vi "KML-Compose2.vi"(0 "TimerIN (sh)":u32, 1 "WriteToFile?":bool, 3 "SPD":string, 4 "path to vi or exe":path, 5 "ALT":string, 6 "HED":string, 7 "Range":string="1500", 9 "Tilt":string="0", 11 "error in":errorcluster, 12 "Current Location":string, 13 "Heading":string="0", 14 "Coords":string) -> (10 "Timer OUT (sh)":u32, 15 "error out":errorcluster)   [LabVIEW 8.6]
panel:
  out "resulting string":string
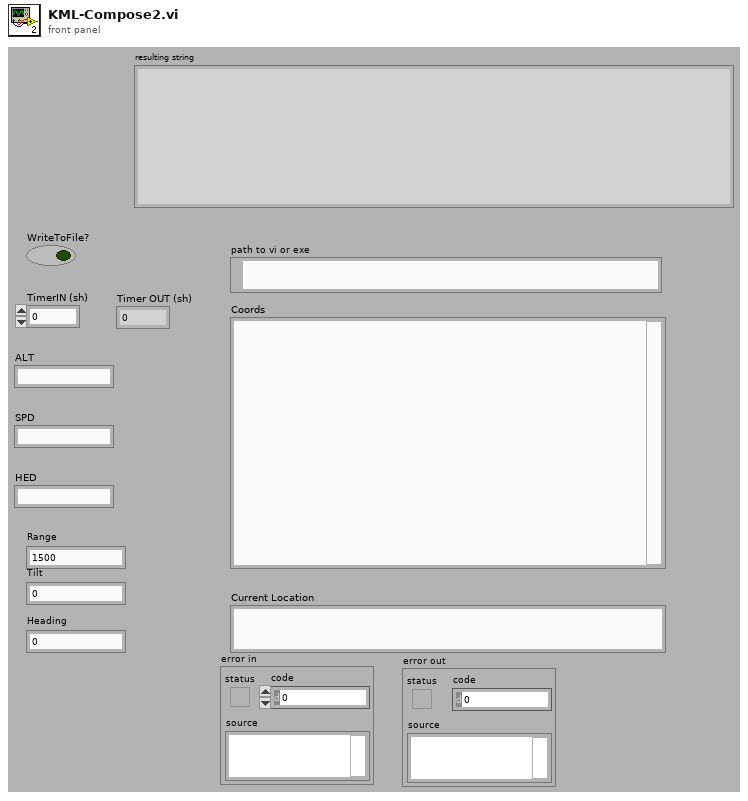
[diagram p1: front panel]
types:
  T1 = enum16{"open", "replace", "create", "open or create", "replace or create", "replace or create with confirmation"}
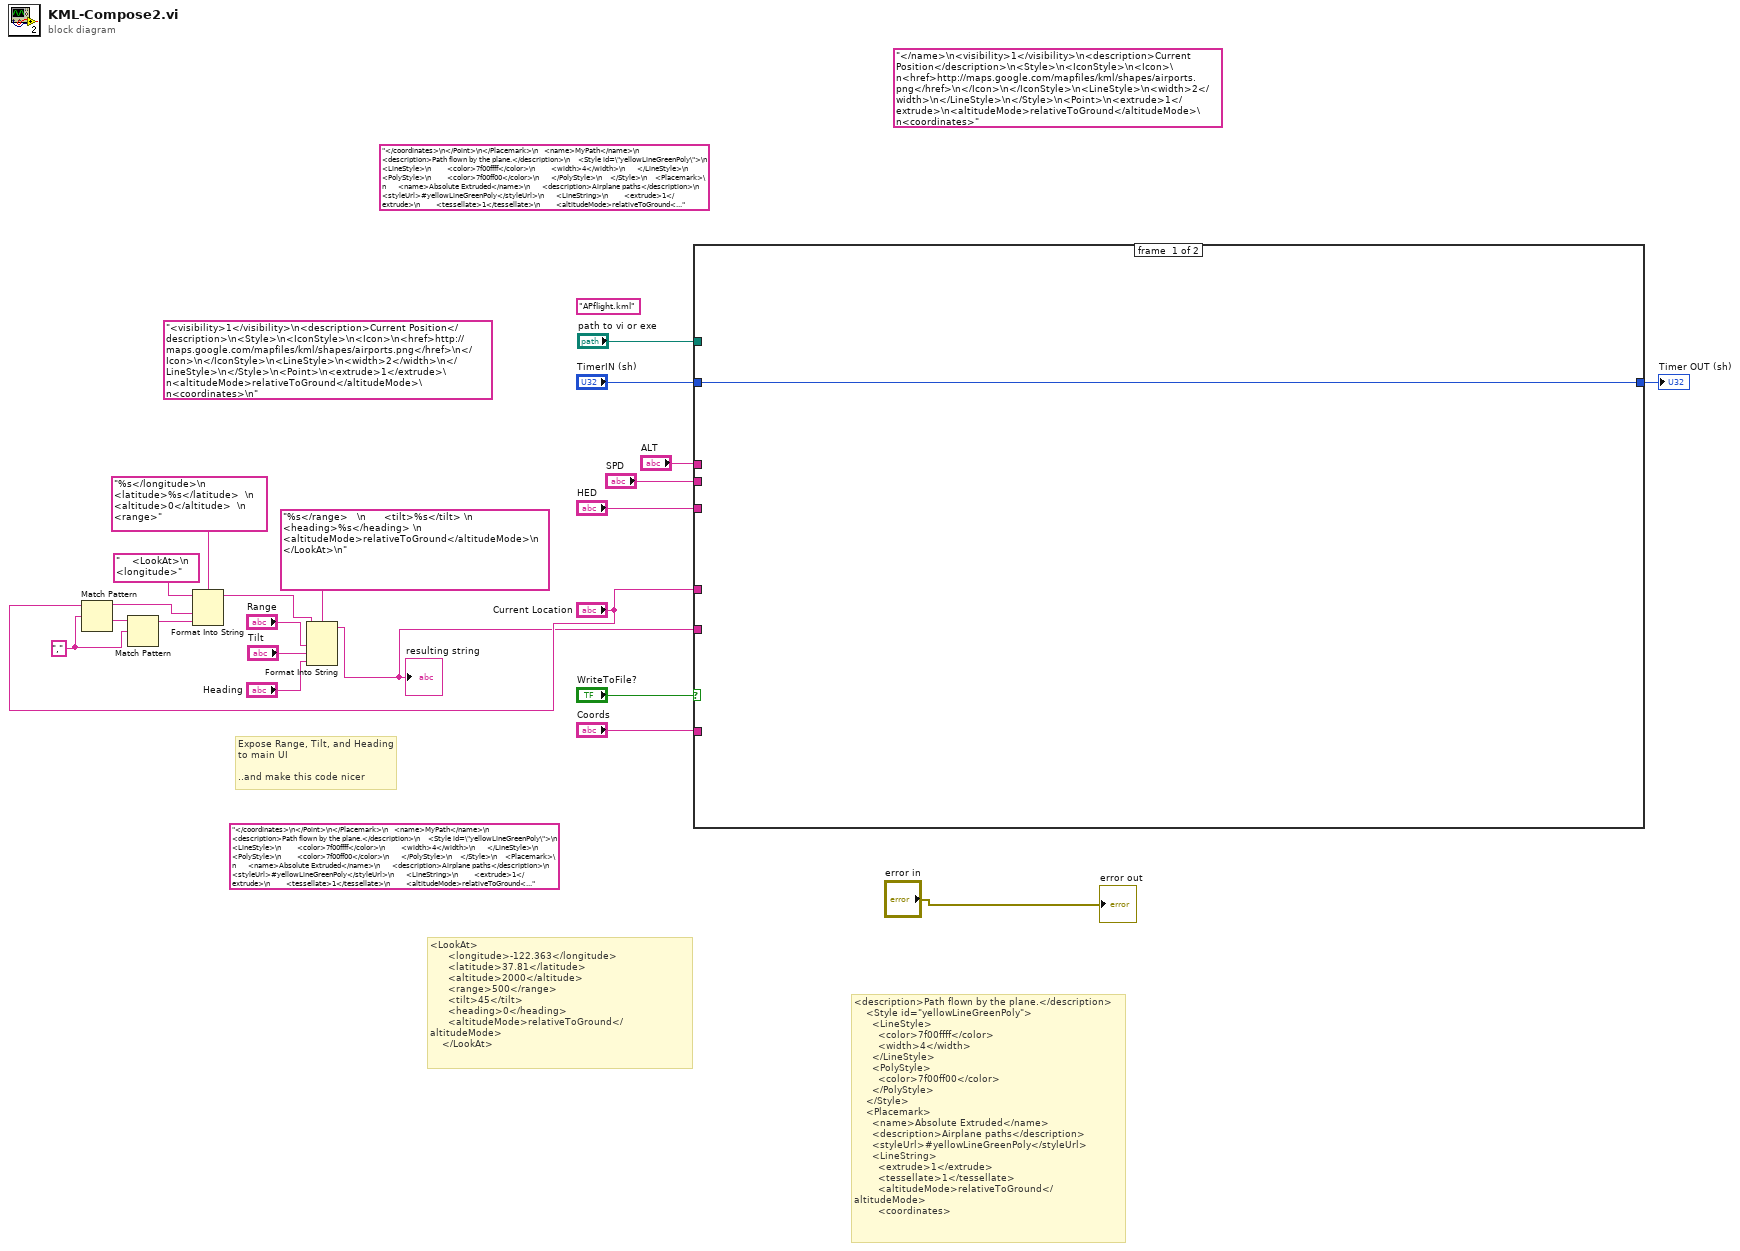
[diagram p0: block diagram]
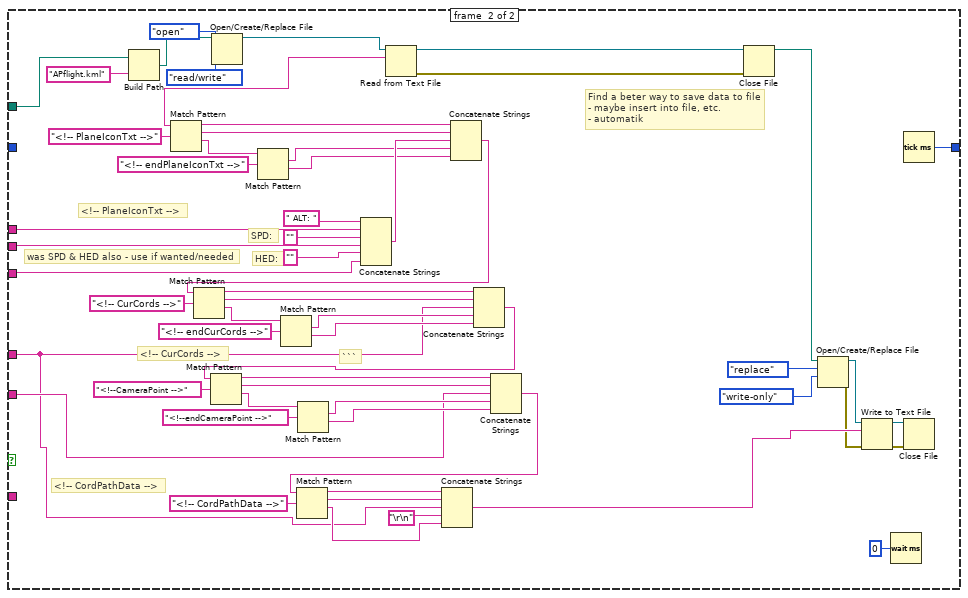
[diagram p2: hidden frame]
diagram:
  (unwired) "APflight.kml" ("name or relative path")
  (unwired) "</name>\n<visibility>1</visibility>\n<description>Current Position</description>\n<Style>\n<IconStyle>\n<Icon>\n<href>http://maps.google.com/mapfiles/kml/shapes/airports.png</href>\n</Icon>\n</IconStyle>\n<LineStyle>\n<width>2</width>\n</LineStyle>\n</Style>\n<Point>\n<extrude>1</extrude>\n<altitudeMode>relativeToGround</altitudeMode>\n<coordinates>"
  (unwired) "</coordinates>\n</Point>\n</Placemark>\n   <name>MyPath</name>\n    <description>Path flown by the plane.</description>\n    <Style id=\"yellowLineGreenPoly\">\n      <LineStyle>\n        <color>7f00ffff</color>\n        <width>4</width>\n      </LineStyle>\n      <PolyStyle>\n        <color>7f00ff00</color>\n      </PolyStyle>\n    </Style>\n    <Placemark>\n      <name>Absolute Extruded</name>\n      <description>Airplane paths</description>\n      <styleUrl>#yellowLineGreenPoly</styleUrl>\n      <LineString>\n        <extrude>1</extrude>\n        <tessellate>1</tessellate>\n        <altitudeMode>relativeToGround</altitudeMode>\n        <coordinates>"
  (unwired) "</coordinates>\n</Point>\n</Placemark>\n   <name>MyPath</name>\n    <description>Path flown by the plane.</description>\n    <Style id=\"yellowLineGreenPoly\">\n      <LineStyle>\n        <color>7f00ffff</color>\n        <width>4</width>\n      </LineStyle>\n      <PolyStyle>\n        <color>7f00ff00</color>\n      </PolyStyle>\n    </Style>\n    <Placemark>\n      <name>Absolute Extruded</name>\n      <description>Airplane paths</description>\n      <styleUrl>#yellowLineGreenPoly</styleUrl>\n      <LineString>\n        <extrude>1</extrude>\n        <tessellate>1</tessellate>\n        <altitudeMode>relativeToGround</altitudeMode>\n        <coordinates>"
  (unwired) "<visibility>1</visibility>\n<description>Current Position</description>\n<Style>\n<IconStyle>\n<Icon>\n<href>http://maps.google.com/mapfiles/kml/shapes/airports.png</href>\n</Icon>\n</IconStyle>\n<LineStyle>\n<width>2</width>\n</LineStyle>\n</Style>\n<Point>\n<extrude>1</extrude>\n<altitudeMode>relativeToGround</altitudeMode>\n<coordinates>\n"
  w2 = "," ("search string/char (-)")
  # "Expose Range, Tilt, and Heading\nto main UI\n\n..and make this code nicer"
  # "<description>Path flown by the plane.</description>\n    <Style id=\"yellowLineGreenPoly\">\n      <LineStyle>\n        <color>7f00ffff</color>\n        <width>4</width>\n      </LineStyle>\n      <PolyStyle>\n        <color>7f00ff00</color>\n      </PolyStyle>\n    </Style>\n    <Placemark>\n      <name>Absolute Extruded</name>\n      <description>Airplane paths</description>\n      <styleUrl>#yellowLineGreenPoly</styleUrl>\n      <LineString>\n        <extrude>1</extrude>\n        <tessellate>1</tessellate>\n        <altitudeMode>relativeToGround</altitudeMode>\n        <coordinates>"
  # "<LookAt>\n      <longitude>-122.363</longitude>\n      <latitude>37.81</latitude>  \n      <altitude>2000</altitude>  \n      <range>500</range>   \n      <tilt>45</tilt> \n      <heading>0</heading> \n      <altitudeMode>relativeToGround</altitudeMode>\n    </LookAt>"
  n1 = Match Pattern(string="Current Location", regular expression=w2) -> (before substring=w11:string, after substring=w13:string)  [unwired: 1 in, 2 out]
  n2 = Match Pattern(string=w13, regular expression=w2) -> (before substring=w12:string)  [unwired: 1 in, 3 out]
  n3 = Format Into String(format string="%s</longitude>\n      <latitude>%s</latitude>  \n      <altitude>0</altitude>  \n       <range>", initial string="    <LookAt>\n      <longitude>", w11, w12) -> (resulting string=w4:string)  [unwired: 1 in, 1 out]
  n4 = Format Into String(format string="%s</range>   \n      <tilt>%s</tilt> \n      <heading>%s</heading> \n      <altitudeMode>relativeToGround</altitudeMode>\n    </LookAt>\n" ("initial string"), initial string=w4, "Range", "Tilt", "Heading") -> (resulting string=w1:string)  [unwired: 1 in, 1 out]
  "resulting string" <- w1
  n5 = case shown="True" "WriteToFile?" {
    tunnel: "ALT" -> [_ w76]
    tunnel: "SPD" -> [_ w75]
    tunnel: "HED" -> [_ w74]
    tunnel: "Current Location" -> [_ w24]
    tunnel: "Coords" -> [_ _]
    tunnel: [w23 w73] -> w20
    tunnel: "TimerIN (sh)" -> [w23 _]
    tunnel: "path to vi or exe" -> [_ w39]
    tunnel: w1 -> [_ w46]
    frame #0 {
    }
    frame #1 {
      # "Find a beter way to save data to file\n- maybe insert into file, etc. \n- automatik"
      # "```"
      # "<!-- CordPathData -->"
      # "<!-- PlaneIconTxt -->"
      # "<!-- CurCords -->"
      # "was SPD & HED also - use if wanted/needed"
      # "HED:"
      # "SPD:"
      n6 = Build Path(base path=w39, name or relative path="APflight.kml") -> (appended path=w34:path)
      n7 = Open/Create/Replace File(file path (use dialog)=w34, operation (0:open)=T1."open", access (0:read/write)=enum16{"read/write", "read-only", "write-only"}."read/write") -> (refnum out=w36:refnum<file>)  [unwired: 3 in, 2 out]
      n8 = Concatenate Strings(" ALT: ", w76, "", w75, "", w74) -> (w67:string)
      n9 = Read from Text File(file (use dialog)=w36) -> (refnum out=w33:refnum<file>, text=w40:string, error out=w32:errorcluster)  [unwired: 3 in, 1 out]
      n10 = Match Pattern(string=w40, regular expression="<!-- PlaneIconTxt -->") -> (before substring=w71:string, match substring=w72:string, after substring=w69:string)  [unwired: 1 in, 1 out]
      n11 = Match Pattern(string=w69, regular expression="<!-- endPlaneIconTxt -->") -> (match substring=w66:string, after substring=w65:string)  [unwired: 1 in, 2 out]
      n12 = Concatenate Strings(w71, w72, w67, w66, w65) -> (w57:string)
      n13 = Match Pattern(string=w57, regular expression="<!-- CurCords -->") -> (before substring=w63:string, match substring=w64:string, after substring=w61:string)  [unwired: 1 in, 1 out]
      n14 = Match Pattern(string=w61, regular expression="<!-- endCurCords -->") -> (match substring=w59:string, after substring=w58:string)  [unwired: 1 in, 2 out]
      n15 = Concatenate Strings(w63, w64, w24, w59, w58) -> (w43:string)
      n16 = Match Pattern(string=w43, regular expression="<!--CameraPoint -->") -> (before substring=w55:string, match substring=w56:string, after substring=w53:string)  [unwired: 1 in, 1 out]
      n17 = Match Pattern(string=w53, regular expression="<!--endCameraPoint -->") -> (match substring=w51:string, after substring=w50:string)  [unwired: 1 in, 2 out]
      n18 = Concatenate Strings(w55, w56, w46, w51, w50) -> (w42:string)
      n19 = Match Pattern(string=w42, regular expression="<!-- CordPathData -->") -> (before substring=w48:string, match substring=w47:string, after substring=w44:string)  [unwired: 1 in, 1 out]
      n20 = Concatenate Strings(w48, w47, w24, "\r\n", w44) -> (w41:string)
      n21 = Close File(refnum=w33, error in=w32) -> (path=w29:path)  [unwired: 1 out]
      n22 = Open/Create/Replace File(file path (use dialog)=w29, operation (0:open)=T1."replace", access (0:read/write)=enum16{"read/write", "read-only", "write-only"}."write-only") -> (refnum out=w28:refnum<file>, error out=w27:errorcluster)  [unwired: 3 in, 1 out]
      n23 = Write to Text File(file (use dialog)=w28, text=w41, error in=w27) -> (refnum out=w80:refnum<file>, error out=w35:errorcluster)  [unwired: 2 out]
      n24 = Wait (ms)(milliseconds to wait=u32 0) -> ()  [unwired: 1 out]
      n25 = Tick Count (ms)() -> (millisecond timer value=w73:u32)
      n26 = Close File(refnum=w80, error in=w35) -> ()  [unwired: 2 out]
    }
  }
  "Timer OUT (sh)" <- w20
  "error out" <- "error in"
